vi "local_variables.vi"() -> ()   [LabVIEW 2018]
panel:
  out "State":string
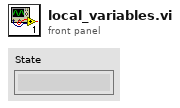
[diagram p1: front panel]
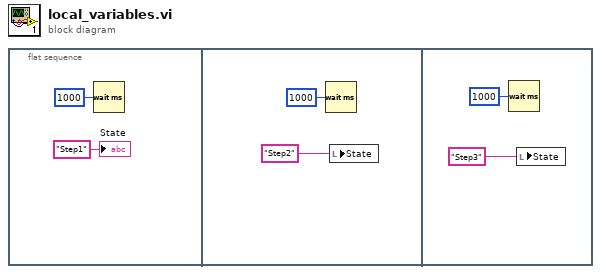
[diagram p0: block diagram]
diagram:
  n1 = flat-sequence {
    frame #0 {
      n2 = Wait (ms)(milliseconds to wait=u32 1000) -> ()  [unwired: 1 out]
      "State" <- "Step1" ("State")
    }
    frame #1 {
      n3 = Wait (ms)(milliseconds to wait=u32 1000) -> ()  [unwired: 1 out]
      n4 = local write "State"("Step2" ("State")) -> ()
    }
    frame #2 {
      n5 = Wait (ms)(milliseconds to wait=u32 1000) -> ()  [unwired: 1 out]
      n6 = local write "State"("Step3" ("State")) -> ()
    }
  }
